vi "micron_setup.vi"(3 "Error in":errorcluster) -> (0 "Error out":errorcluster, 1 "Micron config":T1, 2 "Network error out":errorcluster)   [LabVIEW 2014]
uses:
  micron_config.ctl
  manipulator/squiggle/Host/i2c_interface.ctl
  manipulator/squiggle/Host/fpga_reference.ctl
  testing/Micron params.ctl
  testing/stimulus.ctl
  testing/injection_point.ctl
  filtering/goal_loop_parms.ctl
  testing/mode_conrols.ctl
  testing/manipulator_cal.ctl
  asap/labview/testing/probe_calibration.ctl
  host/network_params.ctl
  cancellation/sq_control_params.ctl
  cancellation/decoupled_gain.ctl
  cancellation/estimation_controls.ctl
  testing/probe_point.ctl
  <vilib>/Utility/error.llb/DialogType.ctl
  <vilib>/DAQmx/create/channels.llb/DAQmx Create Channel (AO-Voltage-Basic).vi
  asap/labview/initialization/globals.vi
  <vilib>/DAQmx/configure/timing.llb/DAQmx Timing (Sample Clock).vi
  <vilib>/DAQmx/create/channels.llb/DAQmx Create Channel (AI-Voltage-Basic).vi
  <vilib>/DAQmx/create/timing.llb/DAQmx Create Timing Source (Control Loop From Task).vi
  <vilib>/DAQmx/create/channels.llb/DAQmx Create Channel (DO-Digital Output).vi
  <vilib>/DAQmx/create/channels.llb/DAQmx Create Channel (DI-Digital Input).vi
  micron_globals.vi
  <resource>/objmgr/daqmx.rc
panel:
  out "Network error message":string
  in  "Extra data range":dbl=10.0
  # "Network errors aren't propagated out to the normal \"Error out\" because getting ignorable \"already bound\" errors is a common problem which causes initialization to fail.  So if you care, the network errors are available here."
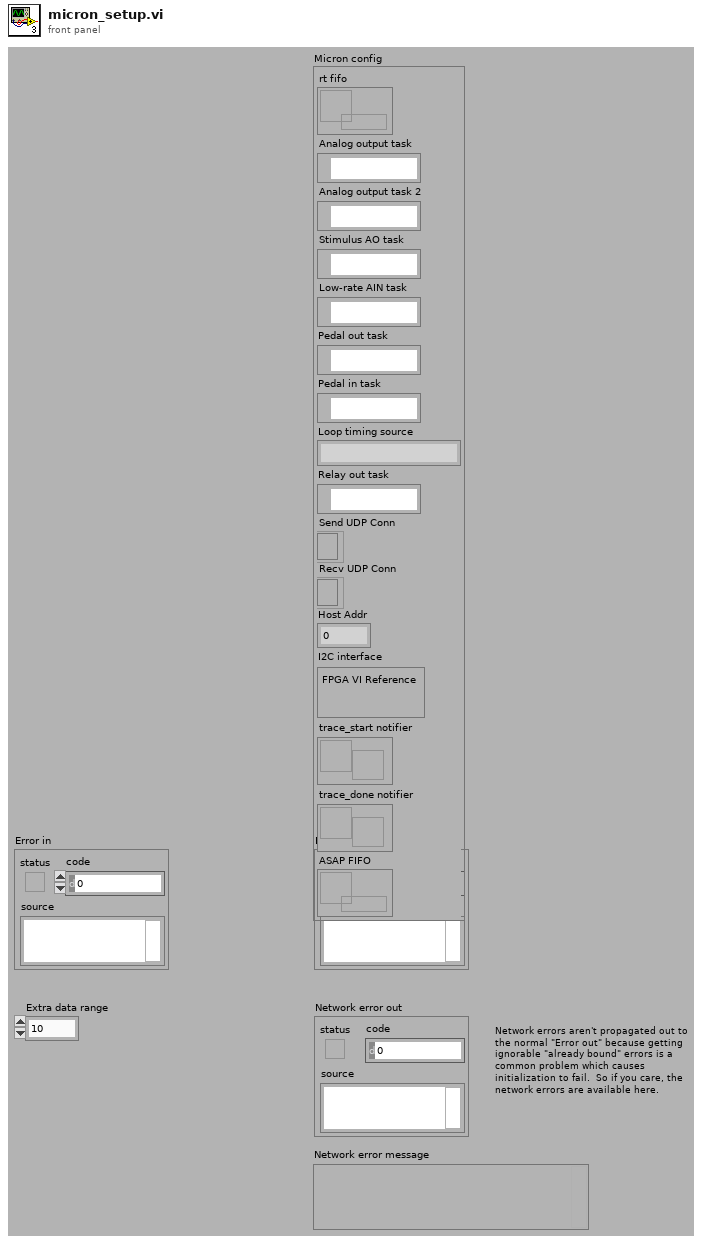
[diagram p1: front panel]
types:
  T1 = typedef "micron_config.ctl" = cluster{"rt fifo":refnum<k33>, "Analog output task":refnum<k21>, "Analog output task 2":refnum<k21>, "Stimulus AO task":refnum<k21>, "Low-rate AIN task":refnum<k21>, "Pedal out task":refnum<k21>, "Pedal in task":refnum<k21>, "Loop timing source":string, "Relay out task":refnum<k21>, "Send UDP Conn":refnum<k16>, "Recv UDP Conn":refnum<k16>, "Host Addr":u32, "I2C interface":T2, "trace_start notifier":refnum<notifier>, "trace_done notifier":refnum<notifier>, "ASAP FIFO":refnum<k33>}
  T2 = typedef "i2c_interface.ctl" = cluster{"FPGA VI Reference":T3}
  T3 = typedef "fpga_reference.ctl" = refnum<k20>
  T4 = typedef "DialogType.ctl" = u16
  T5 = typedef "probe_point.ctl" = enum16{"Position (tip)", "Position (RCM)", "Null pos (tip)", "Null pos (RCM)", "V limiter (tip)", "V Limiter (RCM)", "Goal filter (tip)", "Goal filter (RCM)", "Goal force (tip)", "Goal force (RCM)", "Goal (tip)", "Goal (RCM)", "Link pos 0", "Link pos 1", "KF link pos 0", "KF link pos 1", "Link rate 0", "Link rate 1", "Link residue 0", "Link residue 1", "Link goal 0", "Link goal 1", "Rate limit 0", "Rate limit 1", "Link error 0", "Link error 1", "Controller 0", "Controller 1", "Output 0", "Output 1", "Drive 0", "Drive 1", "Stimulus 0", "Stimulus 1", "Trace data 0", "Trace data 1", "Analog data 0", "Analog data 1", "Status flags", "Light 0", "Light 1", "Light 2", "Light 3", "Light 4", "Light 5", "Goal origin", "Goal rotation 0", "Goal rotation 1", "Goal rotation 2", "Output origin", "Output rotation 0", "Output rotation 1", "Output rotation 2", "Handle origin", "Handle rotation 0", "Handle rotation 1", "Handle rotation 2", "Handle position", "Handle velocity", "Handle acceleration", "Handle angles", "Handle angle rates", "Handle pos residue", "Handle angle residue", "Trace length"}
  T6 = cluster{"read mode":enum16{"polling", "blocking"}, "write mode":enum16{"polling", "blocking"}}
  T7 = enum16{"ASAP/Trigger", "ASAP/Finder", "ASAP/Micron", "ASAP/Micron 2", "Micron 6DOF"}
  T8 = typedef "Micron params.ctl" = cluster{"Stimulus":T9, "Goal Filter A":T11, "Mode controls":T12, "Manipulator type":enum16{"Current piezo", "Voltage piezo"}, "Manipulator calibration":T13, "Network":T15, "Goal Filter B":T11, "Cancellation":T16, "Transition time":sgl, "Estimation":T18}
  T9 = typedef "stimulus.ctl" = cluster{"Type":enum16{"Off", "Step", "Sine", "Triangle", "Arbitrary"}, "Phase":dbl, "Amplitude":sgl[], "Injection point":T10, "Closed loop":bool, "Offset":sgl[], "Tip -> world":bool, "Frequency":dbl, "Length":dbl}
  T10 = typedef "injection_point.ctl" = enum16{"Total pose", "V limiter", "Goal ", "Link position", "KF link position", "Inverse kin", "Link goal", "Link error", "Controller", "Output", "Drive", "Light"}
  T11 = typedef "goal_loop_parms.ctl" = cluster{"Speedup max":sgl, "Speedup thresh":sgl, "Speedup nonlin":sgl, "Filters":cluster{"Lower Fc":sgl, "Lower Q":sgl, "Scale factor":sgl, "Upper Fc":sgl, "Upper Q":sgl, "V limit":sgl, "V limit range":sgl}[]}
  T12 = typedef "mode_conrols.ctl" = cluster{"Hold":bool, "Cancellation":bool, "Goal filter":bool, "Trigger":bool}
  T13 = typedef "manipulator_cal.ctl" = cluster{"Tool offsets":sgl[][], "Tip light calibration":T14, "Handle light calibration":T14, "Base pivots":sgl[][], "Output pivots":sgl[][], "Length center":sgl, "Workspace height":sgl[], "Workspace diameter":sgl[], "Linearization":sgl[][], "Stack travel":sgl, "Saturation pos":sgl, "Inverse filters":cluster{"filter structure":enum32{"IIR 2nd Order", "IIR 4th Order"}, "Reverse Coefficients":dbl[], "Forward Coefficients":dbl[]}[]}
  T14 = typedef "probe_calibration.ctl" = sgl[][]
  T15 = typedef "network_params.ctl" = cluster{"Remote Host":string, "Send Status":bool, "Send Port":u16, "Recv Commands":bool, "Recv Port":u16}
  T16 = typedef "sq_control_params.ctl" = cluster{"KP":T17, "KI":sgl, "KD":T17, "Max vel":sgl, "Max acc":sgl, "Int error limit":sgl, "RCM gain":sgl, "Bypass":bool, "Degraded gain":sgl}
  T17 = typedef "decoupled_gain.ctl" = cluster{"XY":sgl, "Rxy":sgl, "Z":sgl, "Rz":sgl}
  T18 = typedef "estimation_controls.ctl" = cluster{"Link":cluster{"Measure noise":dbl[], "Process noise":dbl[], "Alt process noise":dbl[], "Alt turnoff cycles":i32, "Innovation limit":dbl[], "Residue threshold":dbl, "Enable":bool}, "Handle":cluster{"Measure noise":dbl[], "Process noise":dbl[], "State limits":dbl[], "Innovation limit":dbl[], "Prediction Lookahead":sgl, "Enable":bool}}
  T19 = cluster{"rt fifo":refnum<k33>, "task out":refnum<k21>, "task out":refnum<k21>, "task out":refnum<k21>, "task out":refnum<k21>, "task out":refnum<k21>, "task out":refnum<k21>, "timing source out":string, "task out":refnum<k21>, "Send UDP Conn":refnum<k16>, "Recv UDP Conn":refnum<k16>, "Host Addr":u32, "I2C interface":T2, "notifier out":refnum<notifier>, "notifier out":refnum<notifier>, "rt fifo":refnum<k33>}
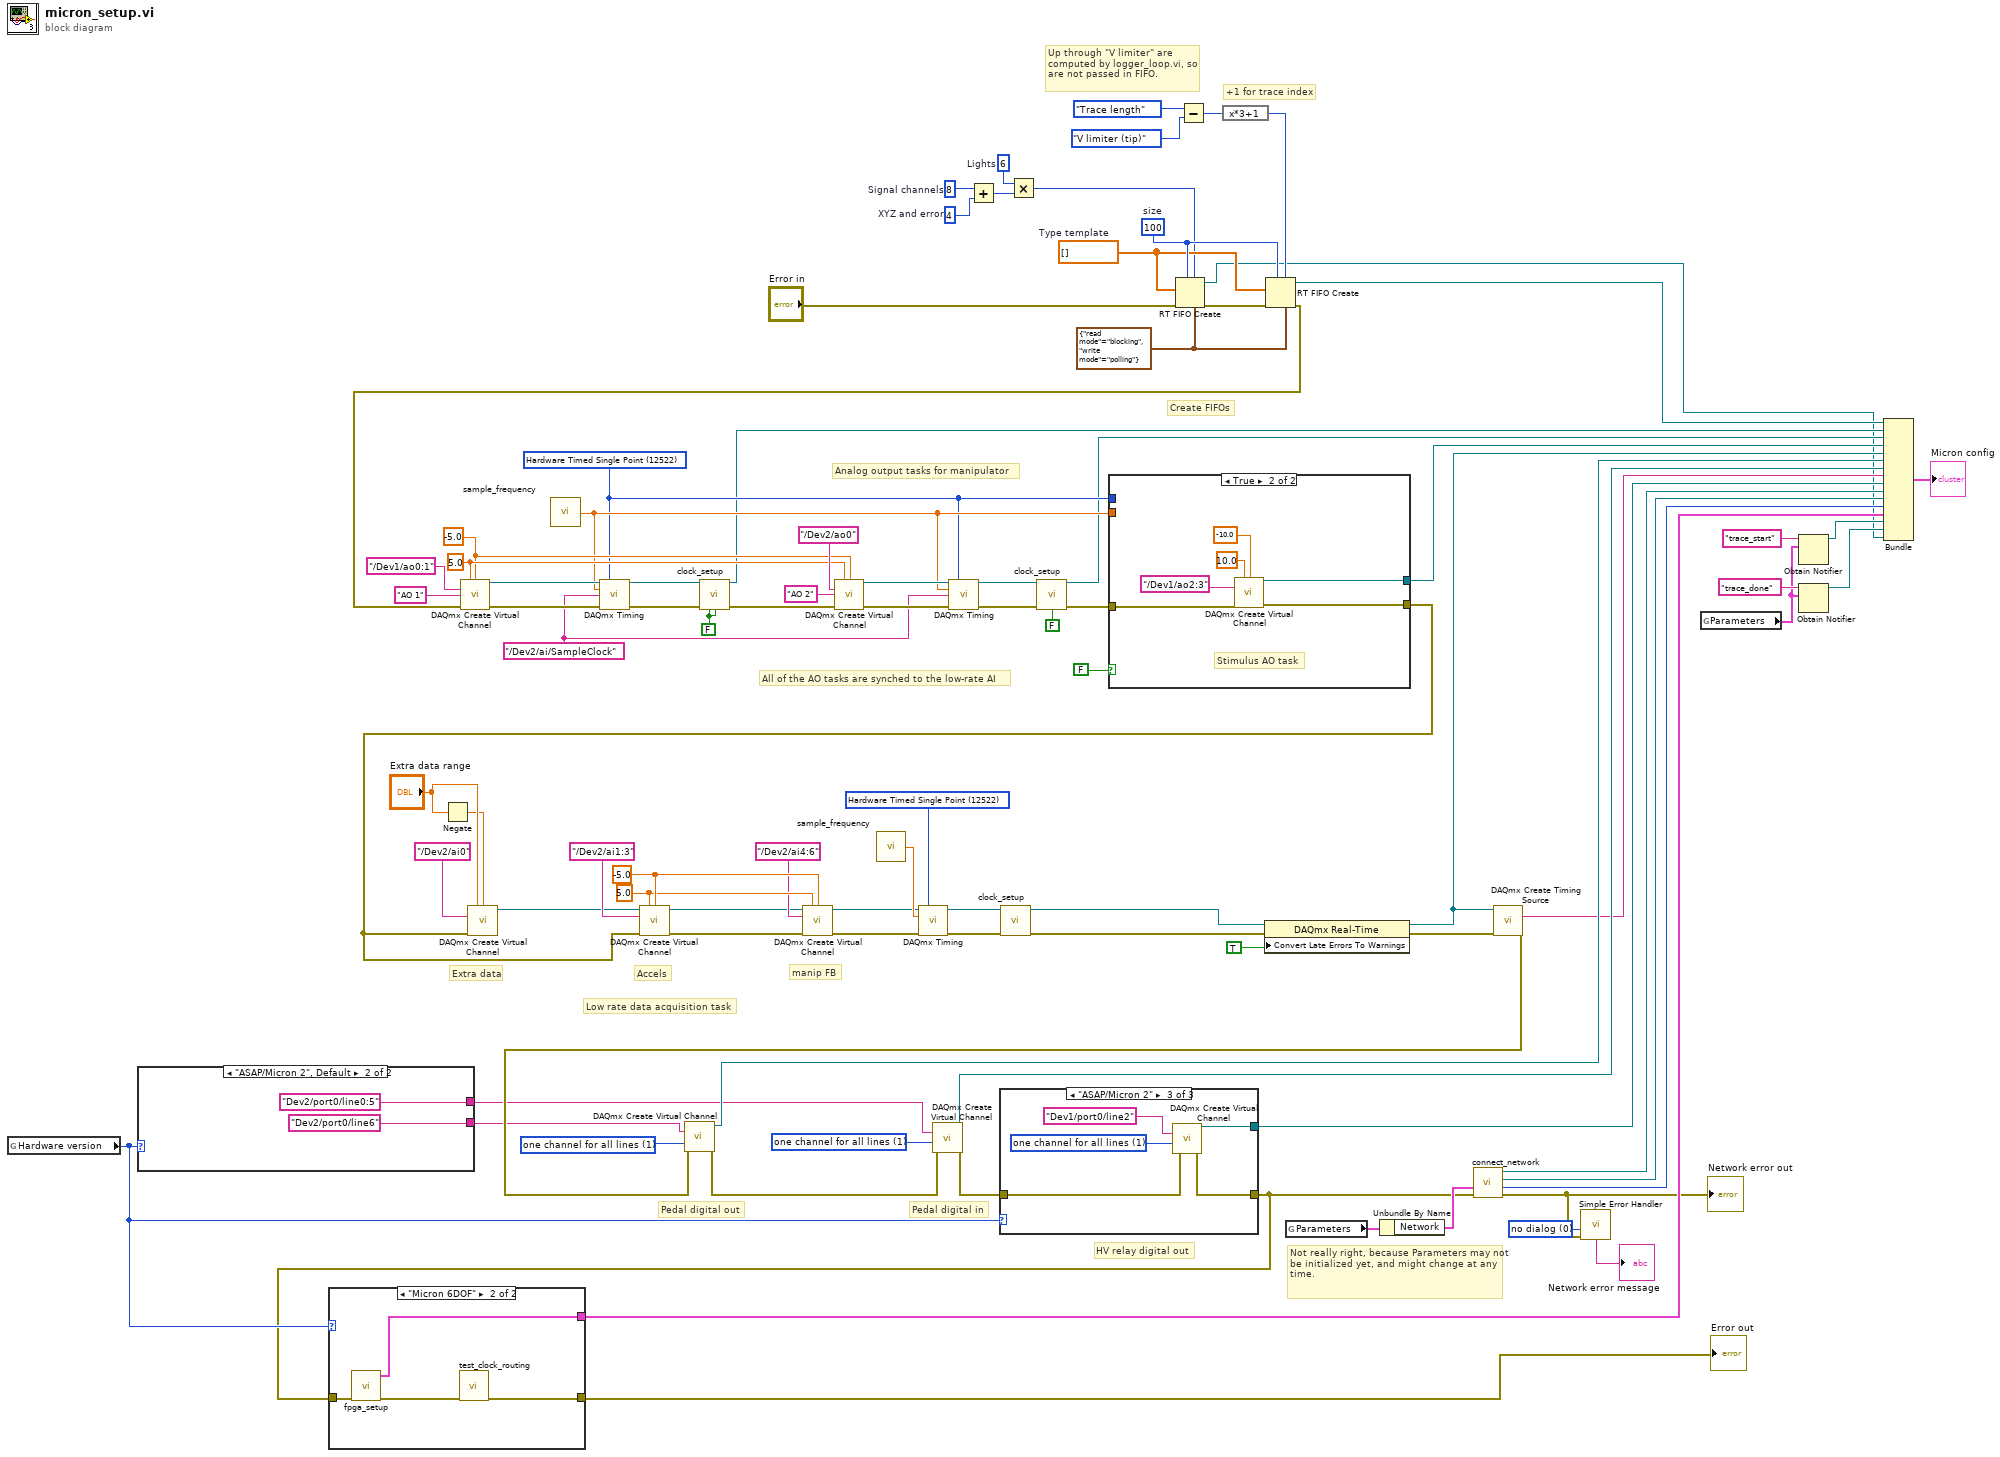
[diagram p0: block diagram]
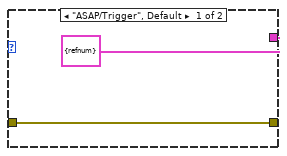
[diagram p2: hidden frame]
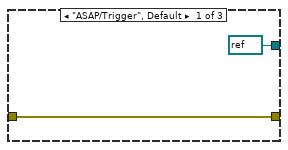
[diagram p3: hidden frame]
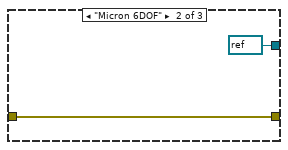
[diagram p4: hidden frame]
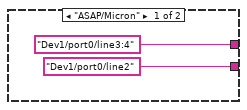
[diagram p5: hidden frame]
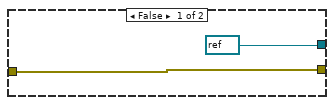
[diagram p6: hidden frame]
diagram:
  w8 = u32 4  # XYZ and error
  w9 = u32 8  # Signal channels
  w6 = u32 6  # Lights
  w23 = T4 0 items=["no dialog", "OK message", "continue or stop message", "OK message + warnings", "continue/stop + warnings"] ("type of dialog (OK msg:1)")
  w28 = FALSE ("Dev2")
  w57 = "/Dev2/ai/SampleClock"
  w58 = 12522 items=["Finite Samples"=10178, "Continuous Samples"=10123, "Hardware Timed Single Point"=12522] ("sample mode")
  w68 = 1 items=["one channel for each line", "one channel for all lines"] ("line grouping")
  w69 = 1 items=["one channel for each line", "one channel for all lines"] ("line grouping")
  w78 = -5.0 ("maximum value")
  w77 = 5.0 ("maximum value")
  w88 = 12522 items=["Finite Samples"=10178, "Continuous Samples"=10123, "Hardware Timed Single Point"=12522] ("sample mode")
  w84 = -5.0 ("minimum value")
  w85 = 5.0 ("maximum value")
  w14 = sgl[] []  # Type template
  w11 = T6 {"read mode"=enum."blocking", "write mode"=enum."polling"} ("r/w modes (polling,polling)")
  w15 = u32 100  # size
  # "Up through \"V limiter\" are computed by logger_loop.vi, so are not passed in FIFO."
  # "+1 for trace index"
  # "Not really right, because Parameters may not be initialized yet, and might change at any time."
  # "HV relay digital out"
  # "Pedal digital in"
  # "All of the AO tasks are synched to the low-rate AI"
  # "Pedal digital out"
  # "manip FB"
  # "Extra data"
  # "Accels"
  # "Low rate data acquisition task"
  # "Analog output tasks for manipulator"
  # "Create FIFOs"
  n1 = global read "globals.vi" "Hardware version"() -> (w41:T7)
  n2 = case shown="\"ASAP/Micron 2\", Default" w41 {
    tunnel: ["Dev1/port0/line2" "Dev2/port0/line6"] -> w51
    tunnel: ["Dev1/port0/line3:4" "Dev2/port0/line0:5"] -> w50
    frame "ASAP/Micron" {
    }
    frame "ASAP/Micron 2", Default {
    }
  }
  n3 = Negate(x="Extra data range") -> (-x=w71:dbl)
  n4 = call "sample_frequency.vi"() -> ("Sample frequency"=w59:dbl)
  n5 = call "sample_frequency.vi"() -> ("Sample frequency"=w76:dbl)
  n6 = Add(x=w9, y=w8) -> (x+y=w7:u32)
  n7 = Multiply(x=w6, y=w7) -> (x*y=w5:u32)
  n8 = RT FIFO Create(1:w14, 3:"Error in", 4:w15, 6:w5, 7:w11) -> (8:w10:refnum<k33>, 11:w13:errorcluster)  [unwired: 2 in, 2 out]
  n9 = Subtract(x=probe_point."Trace length" ("Injection point"), y=probe_point."V limiter (tip)" ("Injection point")) -> (x-y=w38:u16)
  n10 = expression code="x*3+1"(w38) -> (w89:u16)
  n11 = RT FIFO Create(1:w14, 3:w13, 4:w15, 6:w89, 7:w11) -> (8:w92:refnum<k33>, 11:w30:errorcluster)  [unwired: 2 in, 2 out]
  n12 = call-poly <vilib>:"DAQmx Create Virtual Channel.vi"("maximum value"=w85, "minimum value"=w84, "physical channels"="/Dev1/ao0:1", "name to assign"="AO 1", "error in"=w30) -> ("task out"=w64:refnum<k21>, "error out"=w63:errorcluster)  [unwired: 4 in, 5 out]
  n13 = call-poly <vilib>:"DAQmx Timing.vi"("task/channels in"=w64, "sample mode"=w58, "rate"=w59, "source"=w57, "error in"=w63) -> ("task out"=w33:refnum<k21>, "error out"=w34:errorcluster)  [unwired: 2 in, 7 out]
  n14 = call "clock_setup.vi"("task in"=w33, "error in"=w34, "Dev2"=w28, "Set trigger"=w28) -> ("task out"=w32:refnum<k21>, "error out"=w31:errorcluster)  [unwired: 10 in]
  n15 = call-poly <vilib>:"DAQmx Create Virtual Channel.vi"("maximum value"=w85, "minimum value"=w84, "physical channels"="/Dev2/ao0", "name to assign"="AO 2", "error in"=w31) -> ("task out"=w62:refnum<k21>, "error out"=w61:errorcluster)  [unwired: 4 in, 5 out]
  n16 = call-poly <vilib>:"DAQmx Timing.vi"("task/channels in"=w62, "sample mode"=w58, "rate"=w59, "source"=w57, "error in"=w61) -> ("task out"=w36:refnum<k21>, "error out"=w60:errorcluster)  [unwired: 2 in, 7 out]
  n17 = call "clock_setup.vi"("task in"=w36, "error in"=w60, "Set trigger"=FALSE) -> ("task out"=w35:refnum<k21>, "error out"=w80:errorcluster)  [unwired: 11 in]
  n18 = case shown="True" FALSE {
    tunnel: w80 -> [w99 w103]
    tunnel: [refnum<k21> refnum ("task out") w100] -> w91
    tunnel: [w99 w101] -> w4
    tunnel: w59 -> [_ _]
    tunnel: w58 -> [_ _]
    frame False {
    }
    frame True {
      # "Stimulus AO task"
      n19 = call-poly <vilib>:"DAQmx Create Virtual Channel.vi"("maximum value"=10.0, "minimum value"=-10.0, "physical channels"="/Dev1/ao2:3", "error in"=w103) -> ("task out"=w100:refnum<k21>, "error out"=w101:errorcluster)  [unwired: 5 in, 5 out]
    }
  }
  n20 = call-poly <vilib>:"DAQmx Create Virtual Channel.vi"("maximum value"="Extra data range", "minimum value"=w71, "physical channels"="/Dev2/ai0", "error in"=w4) -> ("task out"=w3:refnum<k21>)  [unwired: 5 in, 6 out]
  n21 = call-poly <vilib>:"DAQmx Create Virtual Channel.vi"("task in"=w3, "maximum value"=w77, "minimum value"=w78, "physical channels"="/Dev2/ai1:3", "error in"=w4) -> ("task out"=w2:refnum<k21>, "error out"=w1:errorcluster)  [unwired: 4 in, 5 out]
  n22 = call-poly <vilib>:"DAQmx Create Virtual Channel.vi"("task in"=w2, "maximum value"=w77, "minimum value"=w78, "physical channels"="/Dev2/ai4:6", "error in"=w1) -> ("task out"=w75:refnum<k21>, "error out"=w74:errorcluster)  [unwired: 4 in, 5 out]
  n23 = call-poly <vilib>:"DAQmx Timing.vi"("task/channels in"=w75, "sample mode"=w88, "rate"=w76, "error in"=w74) -> ("task out"=w29:refnum<k21>, "error out"=w81:errorcluster)  [unwired: 3 in, 7 out]
  n24 = call "clock_setup.vi"("task in"=w29, "error in"=w81) -> ("task out"=w26:refnum<k21>, "error out"=w25:errorcluster)  [unwired: 12 in]
  n25 = property class="DAQmx Real-Time"(reference=w26, error in=w25, "Convert Late Errors To Warnings"=TRUE ("ConvLateErrorsToWarnings")) -> (reference out=w53:refnum<k21>, error out=w56:errorcluster)
  n26 = global read "micron_globals.vi" "Parameters"() -> (w45:T8)
  n27 = Unbundle By Name(w45) -> ("Network"=w44:T15)
  n28 = call-poly <vilib>:"DAQmx Create Timing Source.vi"("task/channels in"=w53, "error in"=w56) -> ("timing source out"=w54:string, "error out"=w55:errorcluster)  [unwired: 2 in, 10 out]
  n29 = call-poly <vilib>:"DAQmx Create Virtual Channel.vi"("lines"=w51, "line grouping"=w69, "error in"=w55) -> ("task out"=w67:refnum<k21>, "error out"=w65:errorcluster)  [unwired: 4 in, 7 out]
  n30 = call-poly <vilib>:"DAQmx Create Virtual Channel.vi"("lines"=w50, "line grouping"=w68, "error in"=w65) -> ("task out"=w66:refnum<k21>, "error out"=w52:errorcluster)  [unwired: 2 in, 9 out]
  n31 = case shown="\"ASAP/Micron 2\"" w41 {
    tunnel: w52 -> [w107 w109 w112]
    tunnel: [refnum<k21> refnum ("task out") refnum<k21> refnum ("task out") w111] -> w49
    tunnel: [w107 w109 w110] -> w37
    frame "ASAP/Trigger", Default {
    }
    frame "Micron 6DOF" {
    }
    frame "ASAP/Micron 2" {
      w113 = 1 items=["one channel for each line", "one channel for all lines"] ("line grouping")
      n32 = call-poly <vilib>:"DAQmx Create Virtual Channel.vi"("lines"="Dev1/port0/line2", "line grouping"=w113, "error in"=w112) -> ("task out"=w111:refnum<k21>, "error out"=w110:errorcluster)  [unwired: 2 in, 9 out]
    }
  }
  n33 = case shown="\"Micron 6DOF\"" w41 {
    tunnel: [w116 w117] -> w43
    tunnel: [T2 {"FPGA VI Reference"=refnum} ("I2C interface") w120] -> w42
    tunnel: w37 -> [w116 w119]
    frame "ASAP/Trigger", Default {
    }
    frame "Micron 6DOF" {
      n34 = call "fpga_setup.vi"("error in"=w119) -> ("error out"=w118:errorcluster, "Cluster"=w120:cluster{"FPGA VI Reference Out":T3})  [unwired: 9 in]
      n35 = call "test_clock_routing.vi"("error in (no error)"=w118) -> ("error out"=w117:errorcluster)  [unwired: 10 in]
    }
  }
  "Error out" <- w43
  n36 = call "connect_network.vi"("error in"=w37, "Network params"=w44) -> ("error out"=w24:errorcluster, "Host Addr"=w46:u32, "Recv UDP Conn"=w47:refnum<k16>, "Send UDP Conn"=w48:refnum<k16>)  [unwired: 6 out]
  "Network error out" <- w24
  n37 = call <vilib>:"Simple Error Handler.vi"("type of dialog (OK msg:1)"=w23, "error in (no error)"=w24) -> ("message"=→"Network error message":string)  [unwired: 3 in, 4 out]
  n38 = global read "micron_globals.vi" "Parameters"() -> (w17:T8)
  n39 = Obtain Notifier(name (unnamed)="trace_start", notification data type=w17) -> (notifier out=w19:refnum<notifier>)  [unwired: 2 in, 2 out]
  n40 = Obtain Notifier(name (unnamed)="trace_done", notification data type=w17) -> (notifier out=w18:refnum<notifier>)  [unwired: 2 in, 2 out]
  n41 = Bundle("rt fifo"=w92, "task out"=w32, "task out"=w35, "task out"=w91, "task out"=w53, "task out"=w67, "task out"=w66, "timing source out"=w54, "task out"=w49, "Send UDP Conn"=w48, "Recv UDP Conn"=w47, "Host Addr"=w46, "I2C interface"=w42, "notifier out"=w19, "notifier out"=w18, "rt fifo"=w10) -> (→"Micron config":T19)  [unwired: 1 out]
